vi "sub_Extract_Packets.vi"(6 "Enable?":bool, 7 "Input Complex Samples":cdb[](array[numeric]), 9 "packet_end_loc":i32[](array[numeric]), 11 "packet_start_loc":i32[](array[numeric])) -> (3 "packet_arr":cdb[][](array[numeric]))   [LabVIEW 2015]
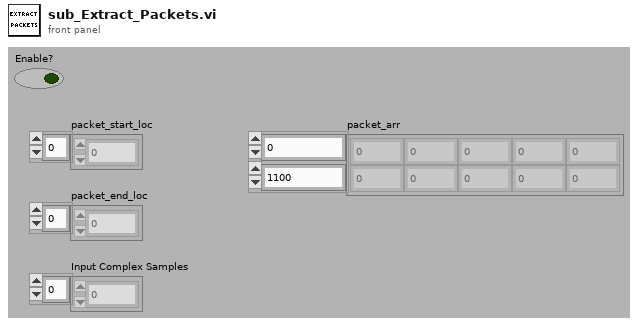
[diagram p1: front panel]
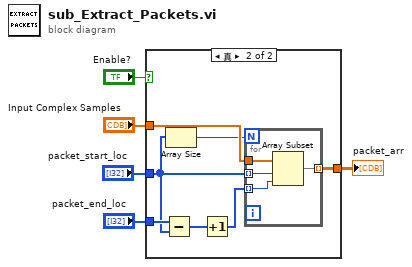
[diagram p0: block diagram]
diagram:
  n1 = case shown="真" "Enable?" {
    tunnel: "packet_end_loc" -> [_ w9]
    tunnel: "packet_start_loc" -> [_ w8]
    tunnel: [_ w12] -> w1
    tunnel: "Input Complex Samples" -> [_ w11]
    frame False {
    }
    frame True {
      n2 = Subtract(x=w9, y=w8) -> (x-y=w7:i32[])
      n3 = Array Size(array=w8) -> (size(s)=w10:i32)
      n4 = Increment(x=w7) -> (x+1=w6:i32[])
      n5 = for {
        N: w10 -> [_]
        tunnel: w11 -> [w16]
        tunnel: w8 -> [w15] mode=indexing
        tunnel: [w14] -> w12 mode=indexing
        tunnel: w6 -> [w13] mode=indexing
        n6 = Array Subset(array=w16, index=w15, length=w13) -> (w14:cdb[])
      }
    }
  }
  "packet_arr" <- w1
